vi "Connection Close.vi"(8 "error in (no error)":errorcluster, 11 "Connection Data In":T1) -> (0 "error out":errorcluster, 3 "Connection Data Out":T1)   [LabVIEW 2014, in "MSX-E3711_dll.lvlib"]
doc: "Cierra la conexión del Web Server."
uses:
  MSX-E3711_dll.lvlib
  Typedef/Connection Data.ctl
  E:/Repositorio Magnis/INF002/v0/Modules/HAL/Drivers/Sync/ADDI-DATA MSX-E3711/API/MSXE371x.dll
  MSXE371x.dll
  E:/Repositorio Magnis/INF002/v0/Modules/HAL/Drivers/Sync/ADDI-DATA MSX-E3711/API/MXCommon.dll
  MXCommon.dll
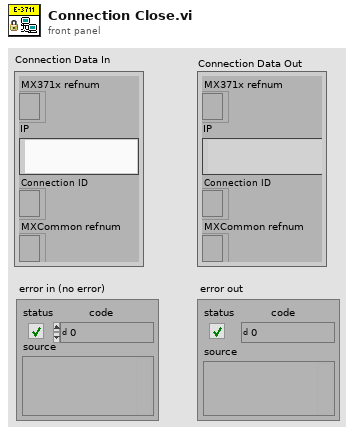
[diagram p1: front panel]
types:
  T1 = typedef "MSX-E3711_dll.lvlib/Connection Data.ctl" = cluster{"MX371x refnum":refnum<k24>, "IP":string, "Connection ID ":refnum<k5>, "MXCommon refnum":refnum<k24>}
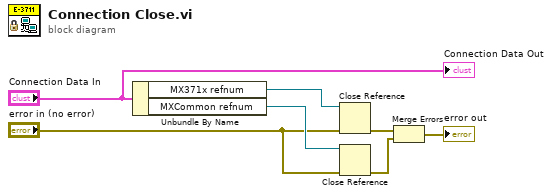
[diagram p0: block diagram]
diagram:
  n1 = Unbundle By Name("Connection Data In") -> ("MX371x refnum"=w7:refnum<k24>, "MXCommon refnum"=w5:refnum<k24>)
  n2 = Close Reference(reference=w7, error in (no error)="error in (no error)") -> (error out=w4:errorcluster)
  n3 = Close Reference(reference=w5, error in (no error)="error in (no error)") -> (error out=w3:errorcluster)
  n4 = Merge Errors(w4, w3) -> (→"error out":errorcluster)
  "Connection Data Out" <- "Connection Data In"
